vi "Example Read BLF.vi"() -> ()   [LabVIEW 2015]
doc: "This is a demo VI to show how the Read Write BLF API works.\n\n-------------\nBrian Hoover (Hooovahh)"
uses:
  Controls/Cluster - CAN Frame.ctl
  Controls/Enum - CAN Data Type.ctl
  Read Write BLF.lvclass/Read Write BLF.ctl
  VIs/Write CAN Frame.vi
  VIs/Set Measurement Start Time.vi
  <vilib>/Utility/error.llb/Error Cluster From Error Code.vi
  Read Write BLF.lvclass
panel:
  out "Object Count":u32
  out "error out":errorcluster
  in  "Frames To Write":T1[](array[typedef])=[{"timestamp"=timestamp(3563447672.613684 s since 1904-01-01), "payload"=[255, 153, 0, 0, 9, 0, 0, 2], "identifier"=134217727, "extended?"=TRUE, "echo?"=FALSE, "type"=2}, {"timestamp"=timestamp(3563447673.7179947 s since 1904-01-01), "payload"=[3, 0, 0, 0, 0, 0, 0], "identifier"=3, "extended?"=FALSE, "echo?"=TRUE, "type"=0}] {"type" items=["CAN Data"=0, "CAN Remote"=1, "CAN Bus Error"=2, "CAN 2.0 Data"=8, "CAN FD Data"=16, "CAN FD+BRS Data"=24, "J1939 Data"=192, "Delay"=224, "Log Trigger"=225, "Start Trigger"=226]; "payload" format="%x"; "timestamp" format="%<%.7X\n%x>T"; "identifier" format="%x"}
  out "Read Frames":T1[](array[typedef]) {"type" items=["CAN Data"=0, "CAN Remote"=1, "CAN Bus Error"=2, "CAN 2.0 Data"=8, "CAN FD Data"=16, "CAN FD+BRS Data"=24, "J1939 Data"=192, "Delay"=224, "Log Trigger"=225, "Start Trigger"=226]; "payload" format="%x"; "timestamp" format="%<%.7X\n%x>T"; "identifier" format="%x"}
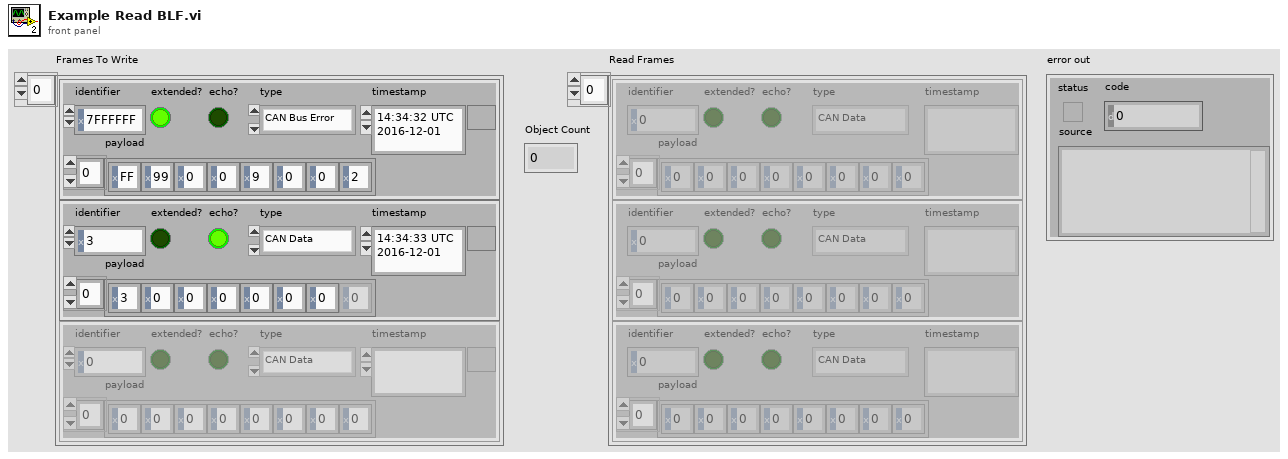
[diagram p1: front panel]
types:
  T1 = typedef "Read Write BLF.lvclass/Cluster - CAN Frame.ctl" = cluster{"timestamp":timestamp, "payload":u8[], "identifier":u32, "extended?":bool, "echo?":bool, "type":T2}
  T2 = typedef "Read Write BLF.lvclass/Enum - CAN Data Type.ctl" = u8
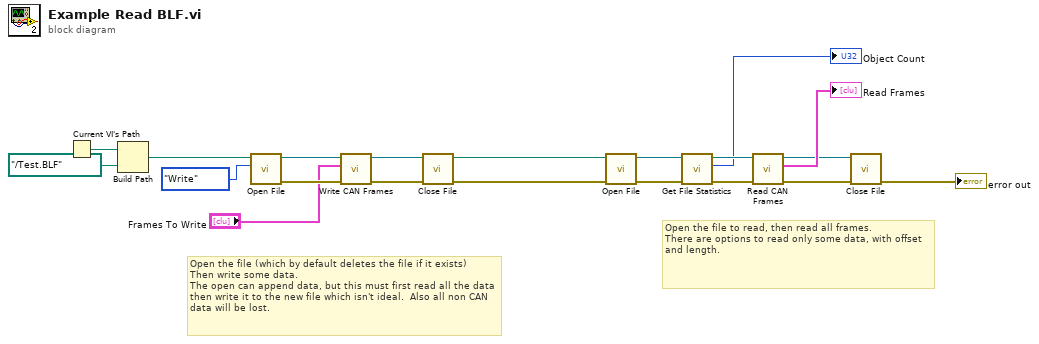
[diagram p0: block diagram]
diagram:
  # "Open the file to read, then read all frames.\nThere are options to read only some data, with offset and length."
  # "Open the file (which by default deletes the file if it exists)\nThen write some data.\nThe open can append data, but this must first read all the data then write it to the new file which isn't ideal.  Also all non CAN data will be lost."
  n1 = Current VI's Path() -> (path=w7:path)
  n2 = Build Path(base path=w7, name or relative path=path "../Test.BLF") -> (appended path=w5:path)
  n3 = call "Open File.vi"("Method (Read)"=enum16{"Write", "Read"}."Write", "Log Path"=w5) -> ("error out"=w15:errorcluster, "BLF File"=w16:refnum<class "Read Write BLF.lvclass">)  [unwired: 8 in]
  n4 = call "Write CAN Frames.vi"("error in (no error)"=w15, "Frames"="Frames To Write", "Read Write BLF in"=w16) -> ("error out"=w10:errorcluster, "Read Write BLF out"=w11:refnum<class "Read Write BLF.lvclass">)  [unwired: 7 in]
  n5 = call "Close File.vi"("error in (no error)"=w10, "BLF File"=w11) -> ("error out"=w12:errorcluster, "BLF Path"=w14:path)  [unwired: 8 in]
  n6 = call "Open File.vi"("error in (no error)"=w12, "Log Path"=w14) -> ("error out"=w13:errorcluster, "BLF File"=w3:refnum<class "Read Write BLF.lvclass">)  [unwired: 8 in]
  n7 = call "Get File Statistics.vi"("error in (no error)"=w13, "Read Write BLF in"=w3) -> ("error out"=w4:errorcluster, "Object Count"=→"Object Count":u32, "Read Write BLF out"=w2:refnum<class "Read Write BLF.lvclass">)  [unwired: 3 in, 4 out]
  n8 = call "Read CAN Frames.vi"("error in (no error)"=w4, "BLF File In"=w2) -> ("error out"=w20:errorcluster, "CAN Frames"=→"Read Frames":T1[], "BLF File Out"=w18:refnum<class "Read Write BLF.lvclass">)  [unwired: 6 in, 1 out]
  n9 = call "Close File.vi"("error in (no error)"=w20, "BLF File"=w18) -> ("error out"=→"error out":errorcluster)  [unwired: 8 in, 1 out]
